vi "SumU8.vi"(1 "Array":u8[](array[numeric])=[0, 0, 0, 0, 0, 0, 0, 0, 0, 0, 0, 0, 0, 0, 0, 0, 0, 0, 0, 0, 0, 0, 0]) -> (0 "Sum":u8)   [LabVIEW 2015]
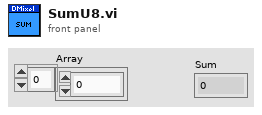
[diagram p1: front panel]
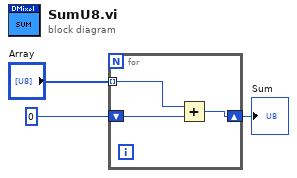
[diagram p0: block diagram]
diagram:
  n1 = for {
    tunnel: "Array" -> [w6] mode=indexing
    shift-right: [w5] -> w1
    shift-left: u8 0 -> [w4]
    n2 = Add(x=w6, y=w4) -> (x+y=w5:u8)
  }
  "Sum" <- w1
